vi "Load New Bitfile.vi"(8 "error in (no error)":errorcluster, 10 "NewVal":path, 11 "Item Ref in":T1 format="%.0x") -> (0 "error out":errorcluster, 3 "Section Ref out":T1 format="%.0x")   [LabVIEW 2016, in "FPGA Addon System Explorer.lvlib"]
uses:
  FPGA Addon System Explorer.lvlib
  <vilib>/NI Veristand/Custom Device API/Custom Device Item Ref.ctl
  Shared/Constants.vi
  <vilib>/NI Veristand/Custom Device API/Set Item Property (Variant).vi
  Shared/FPGA Addon Shared.lvlib
  <vilib>/NI VeriStand/Custom Device API/Custom Device API.lvlib
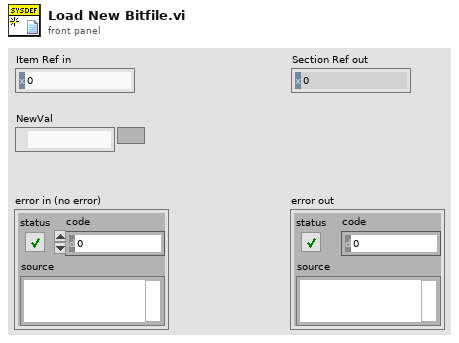
[diagram p1: front panel]
types:
  T1 = typedef "Custom Device API.lvlib/Custom Device Item Ref.ctl" = u64
  T2 = typedef "FPGA Addon System Explorer.lvlib/fpga resource.ctl" = cluster{"name":string, "datatype":string, "channel type":T3, "value":variant, "notes":string}
  T3 = typedef "FPGA Addon System Explorer.lvlib/Channel Type.ctl" = enum16{"Write Channel", "Read Channel", "Write Waveform", "Read Waveform"}
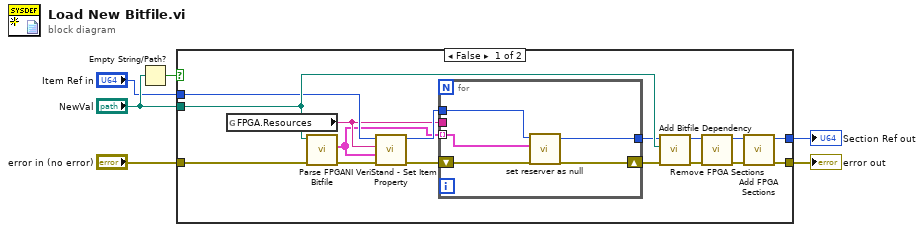
[diagram p0: block diagram]
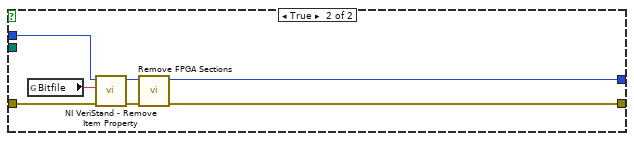
[diagram p2: hidden frame]
diagram:
  n1 = Empty String/Path?(string/path="NewVal") -> (empty?=w4:bool)
  n2 = case shown="False" w4 {
    tunnel: "NewVal" -> [w18 _]
    tunnel: "error in (no error)" -> [w22 w29]
    tunnel: [w14 w34] -> w6
    tunnel: [w13 w33] -> w5
    tunnel: "Item Ref in" -> [w12 w31]
    frame False {
      n3 = global read "Constants.vi" "FPGA.Resources"() -> (w8:string)
      n4 = call "Parse FPGA Bitfile.vi"("error in (no error)"=w22, "Path"=w18) -> ("error out"=w16:errorcluster, "fpga resources"=w7:T2[])  [unwired: 8 in]
      n5 = call-poly <vilib>:"NI VeriStand - Set Item Property.vi"("error in (no error)"=w16, "Value"=w7, "Property Name"=w8, "Item Ref in"=w12) -> ("error out"=w15:errorcluster, "Item Ref out"=w10:T1)  [unwired: 5 in, 1 out]
      n6 = for {
        shift-right: [w26] -> w11
        shift-left: w15 -> [w27]
        tunnel: w8 -> [_]
        tunnel: w7 -> [w23] mode=indexing
        tunnel: w10 -> [w24]
        tunnel: [w25] -> w9
        n7 = call "set reserver as null.vi"("error in (no error)"=w27, "FPGA Resource"=w23, "Item Ref in"=w24) -> ("error out"=w26:errorcluster, "Item Ref out"=w25:T1)  [unwired: 7 in]
      }
      n8 = call "Add Bitfile Dependency.vi"("error in (no error)"=w11, "Path"=w18, "Item Ref in"=w9) -> ("error out"=w19:errorcluster, "Item Ref out"=w17:T1)  [unwired: 7 in]
      n9 = call "Remove FPGA Sections.vi"("error in (no error)"=w19, "Item Ref in"=w17) -> ("error out"=w20:errorcluster, "Item Ref out"=w21:T1)  [unwired: 8 in]
      n10 = call "Add FPGA Sections.vi"("error in (no error)"=w20, "Node Ptr"=w21) -> ("error out"=w14:errorcluster, "Parent Ref out"=w13:T1)  [unwired: 8 in]
    }
    frame True {
      n11 = global read "Constants.vi" "Bitfile"() -> (w32:string)
      n12 = call <vilib>:"NI VeriStand - Remove Item Property.vi"("error in (no error)"=w29, "Property Name"=w32, "Item Ref in"=w31) -> ("error out"=w28:errorcluster, "Item Ref out"=w30:T1)  [unwired: 6 in, 1 out]
      n13 = call "Remove FPGA Sections.vi"("error in (no error)"=w28, "Item Ref in"=w30) -> ("error out"=w34:errorcluster, "Item Ref out"=w33:T1)  [unwired: 8 in]
    }
  }
  "error out" <- w6
  "Section Ref out" <- w5
